vi "Scalar Vector Matrix in 2D.vi"(11 "2D Array":dbl[][](array[numeric])) -> (0 "Is Matrix?":bool, 1 "Is Vector?":bool, 2 "Is Scalar?":bool, 3 "Is Empty?":bool, 4 "Dim Max":i32, 5 "Dimensions":i32[](array[numeric]), 6 "Dim Min":i32)   [LabVIEW 2013]
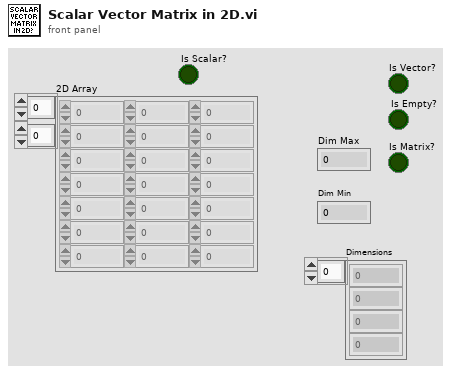
[diagram p1: front panel]
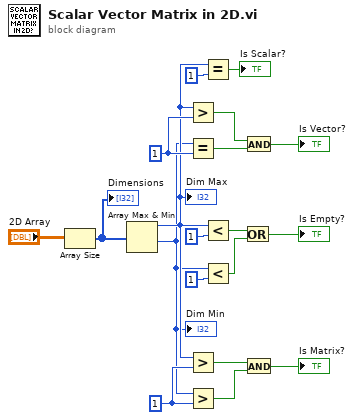
[diagram p0: block diagram]
diagram:
  w8 = 1 ("y")
  w15 = 1 ("y")
  n1 = Array Size(array="2D Array") -> (size(s)=w19:i32[])
  "Dimensions" <- w19
  n2 = Array Max & Min(array=w19) -> (max value=w7:i32, min value=w1:i32)  [unwired: 2 out]
  "Dim Min" <- w1
  "Dim Max" <- w7
  n3 = Greater?(x=w7, y=w15) -> (0:w14:bool)
  n4 = Equal?(x=w1, y=w15) -> (x = y?=w13:bool)
  n5 = Greater?(x=w7, y=w8) -> (0:w9:bool)
  n6 = Greater?(x=w1, y=w8) -> (0:w10:bool)
  n7 = Equal?(x=w7, y=1) -> (x = y?=→"Is Scalar?":bool)
  n8 = Less?(x=w7, y=1) -> (x < y?=w5:bool)
  n9 = Less?(x=w1, y=1) -> (x < y?=w2:bool)
  n10 = Or(x=w5, y=w2) -> (x .or. y?=→"Is Empty?":bool)
  n11 = And(x=w14, y=w13) -> (x .and. y?=→"Is Vector?":bool)
  n12 = And(x=w9, y=w10) -> (x .and. y?=→"Is Matrix?":bool)
